vi "Prime BSI R3 Preview and Capture.vi"(0 "Prime Notifier":refnum<notifier>, 7 "Camera Handle":u32, 11 "Exposure (sec)":dbl=0.1 format="%#_13g", 13 "Image Ref":T1) -> (4 "Prime Notifier (Dup)":refnum<notifier>, 15 "Error":errorcluster)   [LabVIEW 2016]
uses:
  Prime Controls/Prime Notifier Element.ctl
  Prime Controls/Prime Actions.ctl
  Prime Controls/Prime Parameters.ctl
  Prime Controls/Prime Parameter List.ctl
  Prime Controls/Prime ROI.ctl
  <vilib>/vision/Image Controls.llb/IMAQ Image.ctl
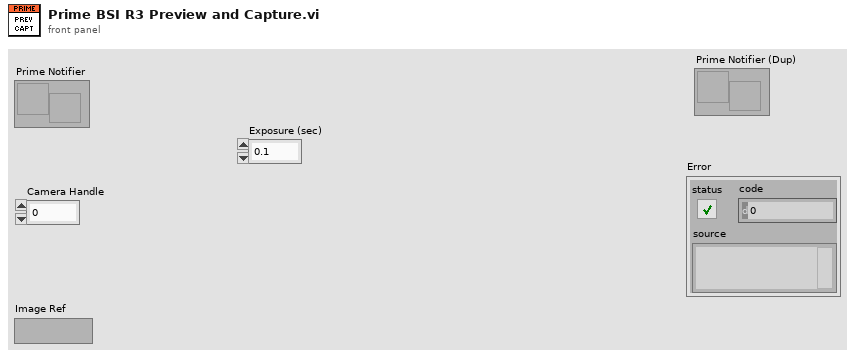
[diagram p1: front panel]
types:
  T1 = typedef "IMAQ Image.ctl" = refnum<image>
  T2 = typedef "Prime Notifier Element.ctl" = cluster{"Prime Actions":T3, "Received?":bool, "Prime Parameter":T4, "Prime ROI":T6, "Running?":bool, "File Path":path, "# of frames":u32, "Image Ref":T1, "Error":errorcluster}
  T3 = typedef "Prime Actions.ctl" = enum16{"Error Check", "Initialize", "Preview", "Record", "Abort", "Record Settings", "Set Parameter", "Get Parameter", "Set ROI", "Get ROI", "Status", "Quit"}
  T4 = typedef "Prime Parameters.ctl" = cluster{"Parameter":T5, "Value":dbl}
  T5 = typedef "Prime Parameter List.ctl" = enum16{"Exposure Time (s)"}
  T6 = typedef "Prime ROI.ctl" = cluster{"X Start":u32, "X End":u32, "X Bin":u32, "Y Start":u32, "Y End":u32, "Y Bin":u32}
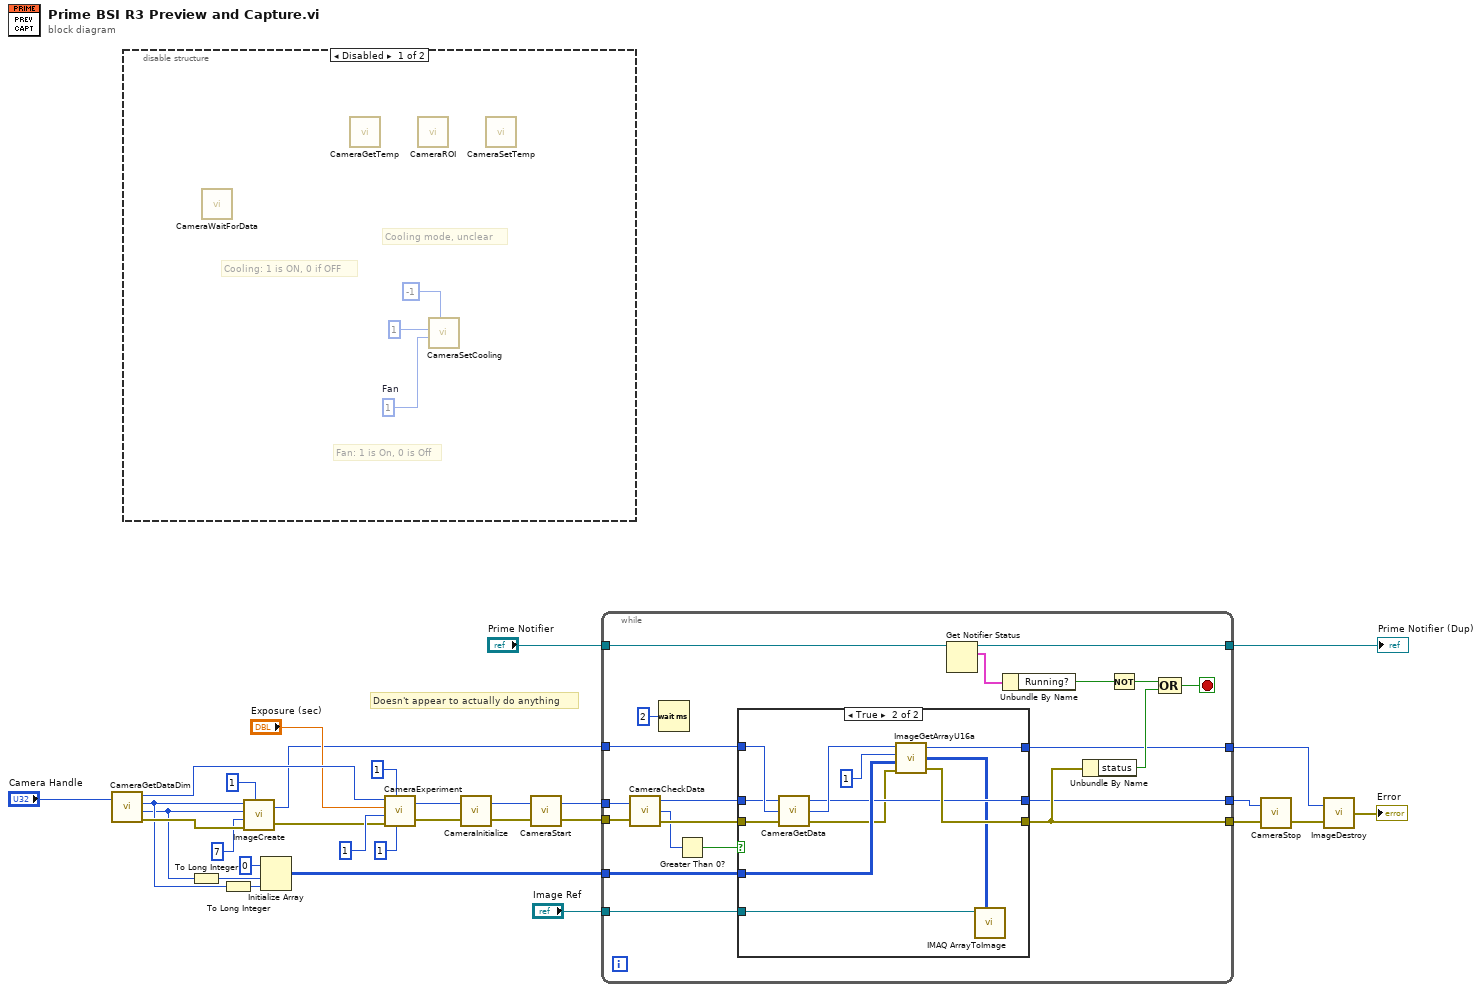
[diagram p0: block diagram]
diagram:
  # "Doesn't appear to actually do anything"
  n1 = call <userlib>:"CameraGetDataDim.vi"("Camera Handle"="Camera Handle") -> ("Camera Handle"=w28:u32, "Xdim"=w5:u32, "Ydim"=w4:u32, "error out"=w31:errorcluster)  [unwired: 1 in]
  n2 = disable-structure shown="Disabled" {
    frame Disabled {
      w33 = 1  # Fan
      # "Cooling mode, unclear"
      # "Cooling: 1 is ON, 0 if OFF"
      # "Fan: 1 is On, 0 is Off"
      n3 = call <userlib>:"CameraWaitForData.vi"() -> ()  [unwired: 4 in, 3 out]
      n4 = call <userlib>:"CameraGetTemp.vi"() -> ()  [unwired: 2 in, 3 out]
      n5 = call <userlib>:"CameraROI.vi"() -> ()  [unwired: 4 in, 2 out]
      n6 = call <userlib>:"CameraSetCooling.vi"("Cooling Mode"=-1, "Fan"=w33, "Cooling"=1) -> ()  [unwired: 3 in, 2 out]
      n7 = call <userlib>:"CameraSetTemp.vi"() -> ()  [unwired: 3 in, 2 out]
    }
    frame Enabled {
    }
  }
  n8 = To Long Integer(number=w4) -> (32bit integer=w18:i32)
  n9 = To Long Integer(number=w5) -> (32bit integer=w17:i32)
  n10 = call <userlib>:"ImageCreate.vi"("X dimension"=w5, "Y dimension"=w4, "Data Type"=u32 7, "error in"=w31, "Number Of Frames"=u32 1) -> ("Image Handle"=w6:u32, "error out"=w3:errorcluster)
  n11 = Initialize Array(u16 0 ("element"), w18, w17) -> (w15:u16[][])
  n12 = call <userlib>:"CameraExperiment.vi"("Number of Accumulations"=u32 1, "Acquire / Focus Flag"=u32 1, "error in"=w3, "Number of Images"=u32 1, "Exposure (sec)"="Exposure (sec)", "Camera Handle"=w28) -> ("error out"=w29:errorcluster, "Camera Handle"=w30:u32)
  n13 = call <userlib>:"CameraInitialize.vi"("error in"=w29, "Camera Handle"=w30) -> ("error out"=w21:errorcluster, "Camera Handle"=w22:u32)
  n14 = call <userlib>:"CameraStart.vi"("error in"=w21, "Camera Handle"=w22) -> ("error out"=w19:errorcluster, "Camera Handle"=w20:u32)
  n15 = while {
    tunnel: w20 -> [w54]
    tunnel: w19 -> [w53]
    tunnel: w6 -> [w38]
    tunnel: w15 -> [w52]
    tunnel: "Prime Notifier" -> [w51]
    tunnel: [w50] -> w13
    tunnel: [w44] -> w12
    tunnel: [w42] -> w10
    tunnel: [w41] -> w9
    tunnel: "Image Ref" -> [w35]
    stop <- w45 stop-if-true
    n16 = call <userlib>:"CameraCheckData.vi"("Camera Handle"=w54, "error in"=w53) -> ("Camera Handle"=w43:u32, "Number Of Frames Available"=w37:i32, "error out"=w48:errorcluster)
    n17 = Wait (ms)(milliseconds to wait=u32 2) -> ()  [unwired: 1 out]
    n18 = Greater Than 0?(x=w37) -> (x > 0?=w36:bool)
    n19 = case shown="True" w36 {
      tunnel: w38 -> [w55 w65]
      tunnel: w52 -> [_ w69]
      tunnel: w48 -> [w57 w63]
      tunnel: [w57 w68] -> w44
      tunnel: [w55 w67] -> w41
      tunnel: [w56 w61] -> w42
      tunnel: w43 -> [w56 w64]
      tunnel: w35 -> [_ w58]
      frame False {
      }
      frame True {
        n20 = call <userlib>:"CameraGetData.vi"("error in"=w63, "Image/Data Handle"=w65, "Camera Handle"=w64) -> ("error out"=w60:errorcluster, "Image/Data Handle"=w62:u32, "Camera Handle"=w61:u32)
        n21 = call <userlib>:"ImageGetArrayU16a.vi"("error in"=w60, "User Array"=w69, "Z position"=u32 1, "Data Handle"=w62) -> ("error out"=w68:errorcluster, "Array uint 16"=w59:u16[][], "Data Handle"=w67:u32)
        n22 = call "IMAQ ArrayToImage"("Image Pixels (U16)"=w59, "Image"=w58) -> ()  [unwired: 8 in, 2 out]
      }
    }
    n23 = Get Notifier Status(notifier=w51) -> (notifier out=w50:refnum<notifier>, current notification=w49:T2)  [unwired: 1 in, 3 out]
    n24 = Unbundle By Name(w49) -> ("Running?"=w47:bool)
    n25 = Unbundle By Name(w44) -> ("status"=w46:bool)
    n26 = Not(x=w47) -> (.not. x?=w40:bool)
    n27 = Compound Arithmetic op=OR(w40, w46) -> (w45:bool)
  }
  "Prime Notifier (Dup)" <- w13
  n28 = call <userlib>:"CameraStop.vi"("error in"=w12, "Camera Handle"=w10) -> ("error out"=w11:errorcluster)  [unwired: 1 out]
  n29 = call <userlib>:"ImageDestroy.vi"("error in"=w11, "Data handle"=w9) -> ("error out"=→"Error":errorcluster)
